vi "Clone.vi"(8 "Error In":errorcluster, 11 "object in":refnum<class "ICloneable.lvclass">) -> (0 "Error Out":errorcluster, 2 "Return(LabVIEW Object)":refnum<class "ICloneable.lvclass">, 3 "object out":refnum<class "ICloneable.lvclass">)   [LabVIEW 2020, in "ICloneable.lvclass"]
doc: "Interface does not need to be marked with the serializable attribute\nMake a new object which is a copy of the object instanced. This object may be either\ndeep copy or a shallow copy depending on the implementation of clone. The default\nObject support for clone does a shallow copy.\nObject Clone()"
uses:
  ICloneable.lvclass
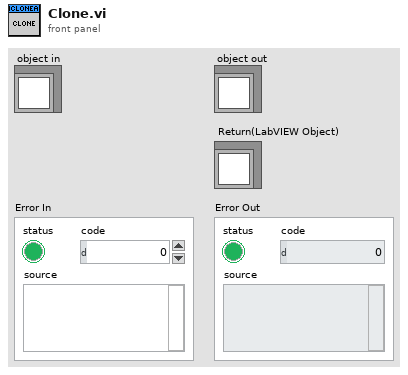
[diagram p1: front panel]
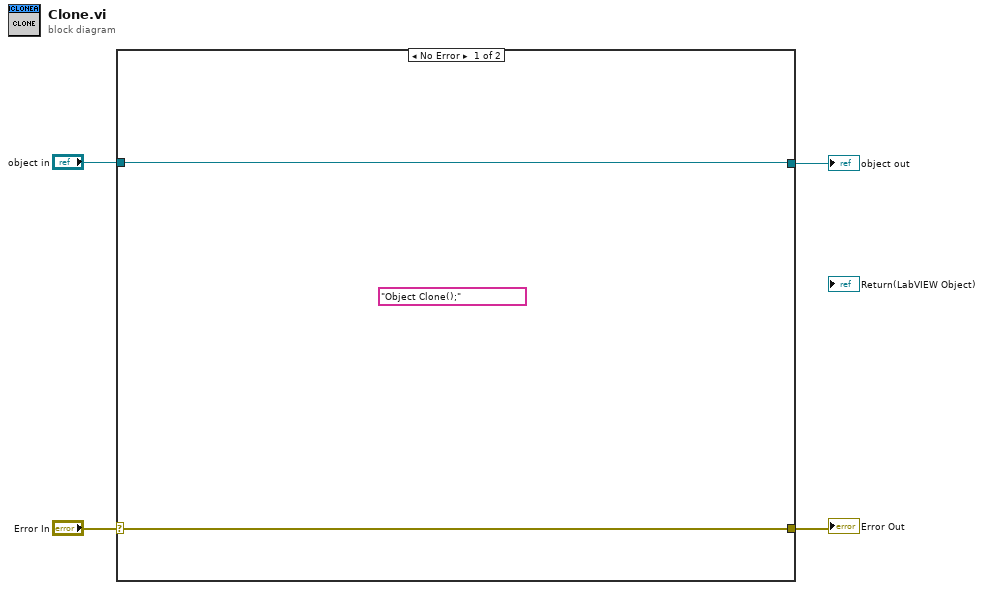
[diagram p0: block diagram]
diagram:
  (unwired) "Object Clone();"
  n1 = case shown="No Error" "Error In" {
    selector: "Error In" -> [w6 w8]
    tunnel: [w6 w8] -> w3
    tunnel: [w5 w7] -> w1
    tunnel: "object in" -> [w5 w7]
    frame No Error {
    }
    frame Error {
    }
  }
  "Error Out" <- w3
  "object out" <- w1
